vi "add line to table.vi"(8 "error in":errorcluster, 10 "line":T1, 11 "operations table":refnum<vi>) -> (0 "error out":errorcluster)   [LabVIEW 2013, in "Scan Engine editor node.lvclass"]
uses:
  Scan Engine editor node.lvclass
  table line.ctl
  <vilib>/NI/Tag Bus Module Framework/channel/TBM channel.lvclass
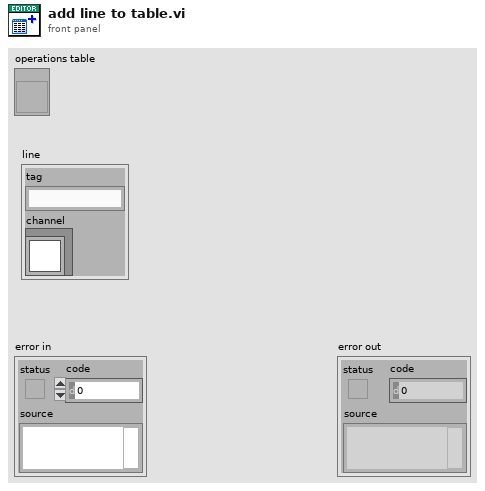
[diagram p1: front panel]
types:
  T1 = typedef "Scan Engine editor node.lvclass/table line.ctl" = cluster{"tag":string, "channel":refnum<class "TBM channel.lvclass">}
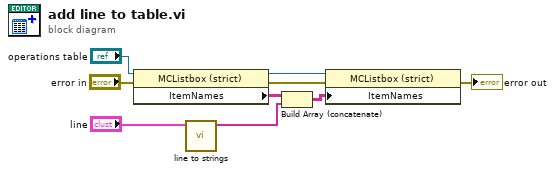
[diagram p0: block diagram]
diagram:
  n1 = property class="MCListbox (strict)"(reference="operations table", error in="error in") -> (reference out=w4:refnum<vi>, error out=w5:errorcluster, "ItemNames"=w6:string[][])
  n2 = call "line to strings.vi"("line"="line") -> ("strings"=w7:string[])  [unwired: 10 in]
  n3 = Build Array (concatenate)(w6, w7) -> (w3:string[][])
  n4 = property class="MCListbox (strict)"(reference=w4, error in=w5, "ItemNames"=w3) -> (error out=→"error out":errorcluster)  [unwired: 1 out]
